vi "HandsRef.vi"(8 "error in (no error)":errorcluster caption="错误输入（无错误）") -> (0 "error out":errorcluster caption="错误输出", 1 "stripped path":path, 3 "簇":T1)   [LabVIEW 2016]
uses:
  Controls/handdata.ctl
  <vilib>/picture/3D Picture Control/Object/Create Object (name).vi
  <vilib>/picture/3D Picture Control/NI_3D Picture Control.lvlib
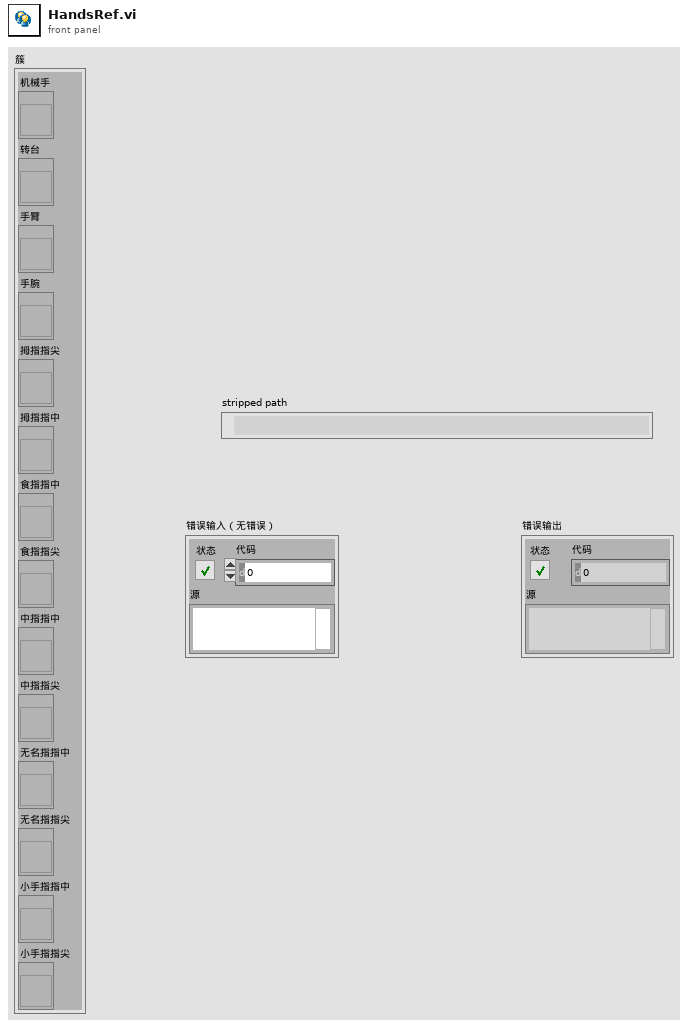
[diagram p1: front panel]
types:
  T1 = typedef "handdata.ctl" = cluster{"机械手":refnum<vi>, "转台":refnum<vi>, "手臂":refnum<vi>, "手腕":refnum<vi>, "拇指指尖":refnum<vi>, "拇指指中 ":refnum<vi>, "食指指中":refnum<vi>, "食指指尖":refnum<vi>, "中指指中":refnum<vi>, "中指指尖":refnum<vi>, "无名指指中":refnum<vi>, "无名指指尖":refnum<vi>, "小手指指中":refnum<vi>, "小手指指尖":refnum<vi>}
  T2 = enum32{"invalid app kind", "Development System", "Run Time System", "Student Edition", "Embedded LabVIEW", "Evaluation", "Custom"}
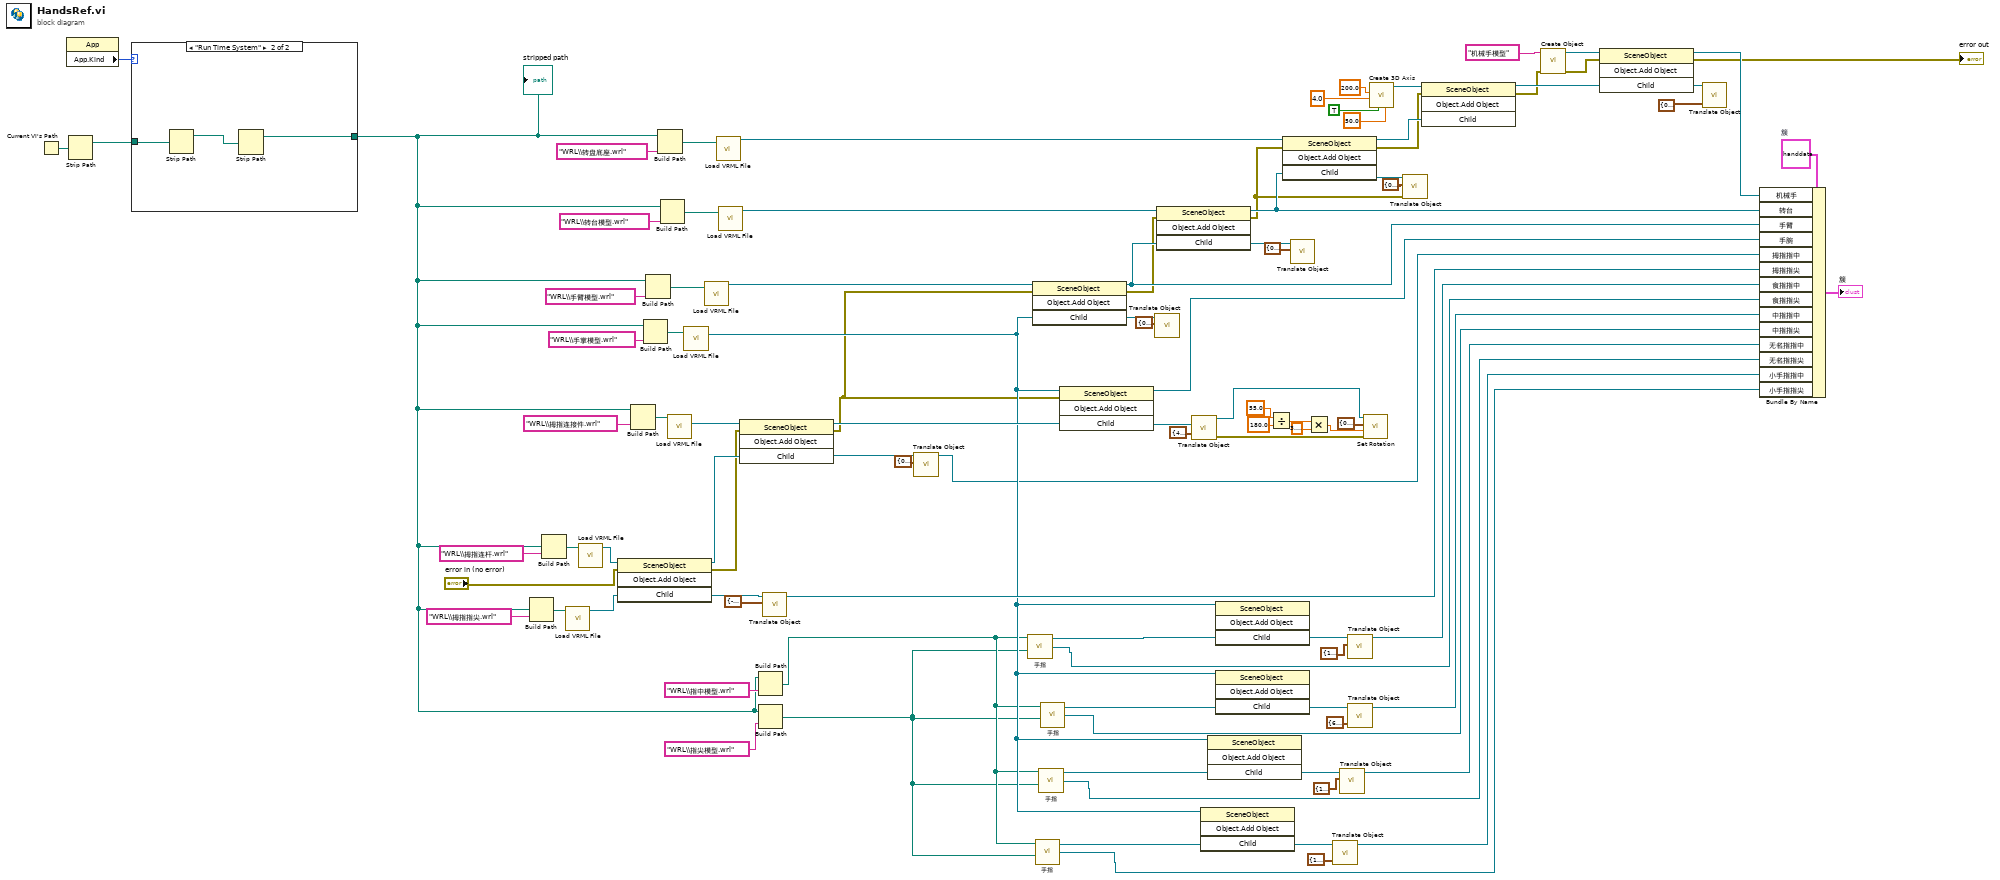
[diagram p0: block diagram]
diagram:
  w98 = T1 {"机械手"=refnum, "转台"=refnum, "手臂"=refnum, "手腕"=refnum, "拇指指尖"=refnum, "拇指指中 "=refnum, "食指指中"=refnum, "食指指尖"=refnum, "中指指中"=refnum, "中指指尖"=refnum, "无名指指中"=refnum, "无名指指尖"=refnum, "小手指指中"=refnum, "小手指指尖"=refnum}  # 簇
  n1 = Current VI's Path() -> (path=w19:path)
  n2 = property class="App"() -> ("App.Kind"=w7:T2)  [unwired: 2 in, 2 out]
  n3 = Strip Path(path=w19) -> (stripped path=w6:path)  [unwired: 1 out]
  n4 = case shown="\"Run Time System\"" w7 {
    tunnel: w6 -> [w100 w101]
    tunnel: [w100 w103] -> w3
    frame "invalid app kind", Default {
    }
    frame "Run Time System" {
      n5 = Strip Path(path=w101) -> (stripped path=w102:path)  [unwired: 1 out]
      n6 = Strip Path(path=w102) -> (stripped path=w103:path)  [unwired: 1 out]
    }
  }
  "stripped path" <- w3
  n7 = Build Path(base path=w3, name or relative path="WRL\\拇指指尖.wrl" ("名称或相对路径")) -> (appended path=w77:path)
  n8 = Build Path(base path=w3, name or relative path="WRL\\拇指连杆.wrl" ("名称或相对路径")) -> (appended path=w59:path)
  n9 = call <vilib>:"Load VRML File.vi"("Path"=w77) -> ("Scene:Read Scene File"=w79:refnum<vi>)  [unwired: 9 in, 1 out]
  n10 = call <vilib>:"Load VRML File.vi"("Path"=w59) -> ("Scene:Read Scene File"=w78:refnum<vi>)  [unwired: 9 in, 1 out]
  n11 = invoke class="SceneObject" method="Object.Add Object"(reference=w78, error in="error in (no error)", "Child"=w79) -> (reference out=w81:refnum<vi>, error out=w10:errorcluster, "Child"=w88:refnum<vi>)  [unwired: 1 in, 1 out]
  n12 = Build Path(base path=w3, name or relative path="WRL\\拇指连接件.wrl" ("名称或相对路径")) -> (appended path=w54:path)
  n13 = Build Path(base path=w3, name or relative path="WRL\\手掌模型.wrl" ("名称或相对路径")) -> (appended path=w43:path)
  n14 = Build Path(base path=w3, name or relative path="WRL\\手臂模型.wrl" ("名称或相对路径")) -> (appended path=w38:path)
  n15 = Build Path(base path=w3, name or relative path="WRL\\转盘底座.wrl" ("名称或相对路径")) -> (appended path=w29:path)
  n16 = Build Path(base path=w3, name or relative path="WRL\\转台模型.wrl" ("名称或相对路径")) -> (appended path=w31:path)
  n17 = call <vilib>:"Load VRML File.vi"("Path"=w54) -> ("Scene:Read Scene File"=w63:refnum<vi>)  [unwired: 9 in, 1 out]
  n18 = call <vilib>:"Load VRML File.vi"("Path"=w43) -> ("Scene:Read Scene File"=w52:refnum<vi>)  [unwired: 9 in, 1 out]
  n19 = call <vilib>:"Load VRML File.vi"("Path"=w38) -> ("Scene:Read Scene File"=w82:refnum<vi>)  [unwired: 9 in, 1 out]
  n20 = call <vilib>:"Load VRML File.vi"("Path"=w29) -> ("Scene:Read Scene File"=w33:refnum<vi>)  [unwired: 9 in, 1 out]
  n21 = call <vilib>:"Load VRML File.vi"("Path"=w31) -> ("Scene:Read Scene File"=w83:refnum<vi>)  [unwired: 9 in, 1 out]
  n22 = invoke class="SceneObject" method="Object.Add Object"(reference=w63, error in=w10, "Child"=w81) -> (reference out=w64:refnum<vi>, error out=w9:errorcluster, "Child"=w61:refnum<vi>)  [unwired: 1 in, 1 out]
  n23 = Build Path(base path=w3, name or relative path="WRL\\指中模型.wrl" ("名称或相对路径")) -> (appended path=w2:path)
  n24 = Build Path(base path=w3, name or relative path="WRL\\指尖模型.wrl" ("名称或相对路径")) -> (appended path=w1:path)
  n25 = call <vilib>:"Translate Object.vi"("Translation"=cluster{"X":sgl, "Y":sgl, "Z":sgl} {"X"=-4.88, "Y"=-2.18, "Z"=28.22}, "Scene.Object In"=w88) -> ("Scene.Object Out"=w90:refnum<vi>)  [unwired: 8 in, 1 out]
  n26 = call <vilib>:"Translate Object.vi"("Translation"=cluster{"X":sgl, "Y":sgl, "Z":sgl} {"X"=0.0, "Y"=0.0, "Z"=-1.67}, "Scene.Object In"=w61) -> ("Scene.Object Out"=w8:refnum<vi>)  [unwired: 8 in, 1 out]
  n27 = call "手指.vi"("指中"=w2, "指尖"=w1) -> ("手指"=w73:refnum<vi>, "指尖"=w91:refnum<vi>)  [unwired: 5 in]
  n28 = invoke class="SceneObject" method="Object.Add Object"(reference=w82, error in=w9, "Child"=w52) -> (reference out=w86:refnum<vi>, error out=w13:errorcluster, "Child"=w41:refnum<vi>)  [unwired: 1 in, 1 out]
  n29 = call "手指.vi"("指中"=w2, "指尖"=w1) -> ("手指"=w71:refnum<vi>, "指尖"=w97:refnum<vi>)  [unwired: 5 in]
  n30 = call "手指.vi"("指中"=w2, "指尖"=w1) -> ("手指"=w72:refnum<vi>, "指尖"=w95:refnum<vi>)  [unwired: 5 in]
  n31 = call "手指.vi"("指中"=w2, "指尖"=w1) -> ("手指"=w75:refnum<vi>, "指尖"=w93:refnum<vi>)  [unwired: 5 in]
  n32 = invoke class="SceneObject" method="Object.Add Object"(reference=w52, error in=w9, "Child"=w64) -> (reference out=w87:refnum<vi>, "Child"=w56:refnum<vi>)  [unwired: 1 in, 2 out]
  n33 = call <vilib>:"Translate Object.vi"("Translation"=cluster{"X":sgl, "Y":sgl, "Z":sgl} {"X"=0.0, "Y"=0.0, "Z"=175.0}, "Scene.Object In"=w41) -> ()  [unwired: 8 in, 2 out]
  n34 = invoke class="SceneObject" method="Object.Add Object"(reference=w83, error in=w13, "Child"=w86) -> (reference out=w85:refnum<vi>, error out=w12:errorcluster, "Child"=w40:refnum<vi>)  [unwired: 1 in, 1 out]
  n35 = call <vilib>:"Translate Object.vi"("Translation"=cluster{"X":sgl, "Y":sgl, "Z":sgl} {"X"=4.74, "Y"=70.2, "Z"=50.34}, "Scene.Object In"=w56) -> ("error out"=w58:errorcluster, "Scene.Object Out"=w57:refnum<vi>)  [unwired: 8 in]
  n36 = invoke class="SceneObject" method="Object.Add Object"(reference=w52, "Child"=w71) -> ("Child"=w46:refnum<vi>)  [unwired: 2 in, 3 out]
  n37 = invoke class="SceneObject" method="Object.Add Object"(reference=w52, "Child"=w72) -> ("Child"=w47:refnum<vi>)  [unwired: 2 in, 3 out]
  n38 = invoke class="SceneObject" method="Object.Add Object"(reference=w52, "Child"=w73) -> ("Child"=w51:refnum<vi>)  [unwired: 2 in, 3 out]
  n39 = invoke class="SceneObject" method="Object.Add Object"(reference=w52, "Child"=w75) -> ("Child"=w74:refnum<vi>)  [unwired: 2 in, 3 out]
  n40 = Divide(x=sgl 55.0 ("Angle 2"), y=sgl 180.0) -> (x/y=w69:sgl)
  n41 = invoke class="SceneObject" method="Object.Add Object"(reference=w33, error in=w12, "Child"=w85) -> (reference out=w36:refnum<vi>, error out=w14:errorcluster, "Child"=w35:refnum<vi>)  [unwired: 1 in, 1 out]
  n42 = call <vilib>:"Translate Object.vi"("Translation"=cluster{"X":sgl, "Y":sgl, "Z":sgl} {"X"=0.0, "Y"=0.0, "Z"=0.0}, "Scene.Object In"=w40) -> ()  [unwired: 8 in, 2 out]
  n43 = Multiply(x=w69, y=3.141592653589793) -> (x*y=w70:dbl)
  n44 = call <vilib>:"Translate Object.vi"("Translation"=cluster{"X":sgl, "Y":sgl, "Z":sgl} {"X"=16.04, "Y"=-45.0, "Z"=85.07}, "Scene.Object In"=w46) -> ("Scene.Object Out"=w96:refnum<vi>)  [unwired: 8 in, 1 out]
  n45 = call <vilib>:"Translate Object.vi"("Translation"=cluster{"X":sgl, "Y":sgl, "Z":sgl} {"X"=11.04, "Y"=-15.0, "Z"=97.57}, "Scene.Object In"=w47) -> ("Scene.Object Out"=w94:refnum<vi>)  [unwired: 8 in, 1 out]
  n46 = call <vilib>:"Translate Object.vi"("Translation"=cluster{"X":sgl, "Y":sgl, "Z":sgl} {"X"=11.04, "Y"=50.0, "Z"=97.57}, "Scene.Object In"=w51) -> ("Scene.Object Out"=w89:refnum<vi>)  [unwired: 8 in, 1 out]
  n47 = call <vilib>:"Translate Object.vi"("Translation"=cluster{"X":sgl, "Y":sgl, "Z":sgl} {"X"=6.04, "Y"=15.0, "Z"=108.78}, "Scene.Object In"=w74) -> ("Scene.Object Out"=w92:refnum<vi>)  [unwired: 8 in, 1 out]
  n48 = call <vilib>:"Set Rotation.vi"("error in (no error)"=w58, "Angle"=w70, "Axis"=cluster{"X":sgl, "Y":sgl, "Z":sgl} {"X"=0.0, "Y"=1.0, "Z"=0.0}, "Scene Object"=w57) -> ()  [unwired: 6 in, 2 out]
  n49 = call <vilib>:"Create 3D Axis.vi"("Character Size"=sgl 50.0, "Axis label?"=TRUE, "Radius"=sgl 4.0, "Length"=sgl 200.0) -> ("New Object Refnum"=w25:refnum<vi>)  [unwired: 6 in, 1 out]
  n50 = call <vilib>:"Translate Object.vi"("error in (no error)"=w12, "Translation"=cluster{"X":sgl, "Y":sgl, "Z":sgl} {"X"=0.0, "Y"=0.0, "Z"=81.5}, "Scene.Object In"=w35) -> ()  [unwired: 7 in, 2 out]
  n51 = invoke class="SceneObject" method="Object.Add Object"(reference=w25, error in=w14, "Child"=w36) -> (reference out=w30:refnum<vi>, error out=w15:errorcluster)  [unwired: 1 in, 2 out]
  n52 = call-poly <vilib>:"Create Object.vi"("error in (no error)"=w15, "Name"="机械手模型") -> ("error out"=w18:errorcluster, "Scene:New Object"=w26:refnum<vi>)  [unwired: 8 in]
  n53 = invoke class="SceneObject" method="Object.Add Object"(reference=w26, error in=w18, "Child"=w30) -> (reference out=w84:refnum<vi>, error out=→"error out":errorcluster, "Child"=w27:refnum<vi>)  [unwired: 1 in, 1 out]
  n54 = call <vilib>:"Translate Object.vi"("Translation"=cluster{"X":sgl, "Y":sgl, "Z":sgl} {"X"=0.0, "Y"=0.0, "Z"=0.0}, "Scene.Object In"=w27) -> ()  [unwired: 8 in, 2 out]
  n55 = Bundle By Name(cluster=w98, "机械手"=w84, "转台"=w85, "手臂"=w86, "手腕"=w87, "拇指指中"=w8, "拇指指尖"=w90, "食指指中"=w89, "食指指尖"=w91, "中指指中"=w92, "中指指尖"=w93, "无名指指中"=w94, "无名指指尖"=w95, "小手指指中"=w96, "小手指指尖"=w97) -> (→"簇":T1)
